vi "Calibration.vi"() -> ()   [LabVIEW 2023]
uses:
  Communication/PCAN2023/PCAN API.lvlib
panel:
  out "Read Current Offset":bool
  out "Perform Current Offset":bool
  out "Set Manifacturing":bool
  out "Nexteer Connect":bool
  out "error out":errorcluster
  in  "error in":errorcluster
  in  "Channel":u16=81 format="%x"
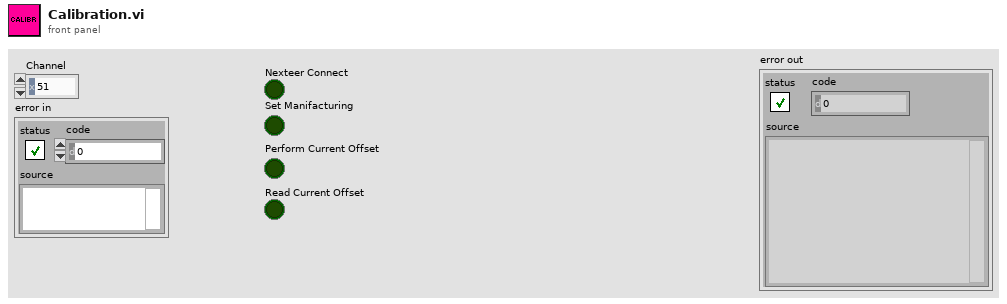
[diagram p1: front panel]
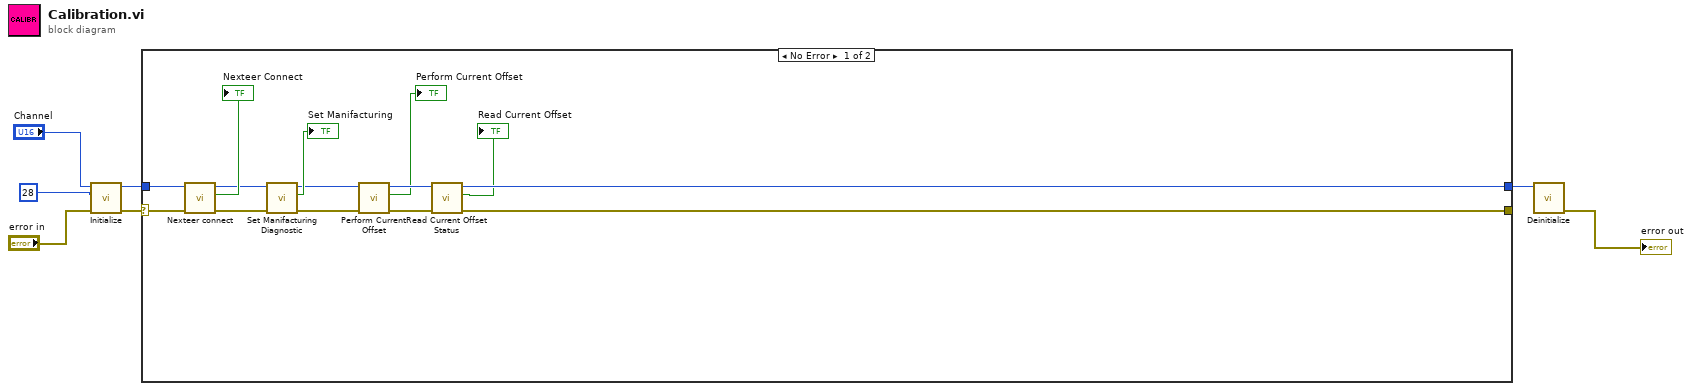
[diagram p0: block diagram]
diagram:
  n1 = call "Initialize.vi"("error in"="error in", "Btr0Btr1"=u16 28, "Channel"="Channel") -> ("error out"=w1:errorcluster, "Channel out"=w4:u16)  [unwired: 6 in, 1 out]
  n2 = case shown="No Error" w1 {
    selector: w1 -> [w20 w23]
    tunnel: w4 -> [w21 w22]
    tunnel: [w11 w22] -> w3
    tunnel: [w10 w23] -> _
    frame No Error {
      n3 = call "Nexteer connect.vi"("error in"=w20, "Channel in"=w21) -> ("error out"=w17:errorcluster, "Pass"=→"Nexteer Connect":bool, "Channel out"=w18:u16)  [unwired: 5 in]
      n4 = call "Set Manifacturing Diagnostic.vi"("error in"=w17, "Channel in"=w18) -> ("error out"=w14:errorcluster, "Pass"=→"Set Manifacturing":bool, "Channel out"=w15:u16)  [unwired: 5 in]
      n5 = call "Perform Current Offset.vi"("error in"=w14, "Channel in"=w15) -> ("error out"=w12:errorcluster, "Pass"=→"Perform Current Offset":bool, "Channel out"=w13:u16)  [unwired: 5 in]
      n6 = call "Read Current Offset Status.vi"("error in"=w12, "Channel in"=w13) -> ("error out"=w10:errorcluster, "Pass"=→"Read Current Offset":bool, "Channel out"=w11:u16)  [unwired: 5 in]
    }
    frame Error {
    }
  }
  n7 = call "Deinitialize.vi"("Channel"=w3) -> ("error out"=→"error out":errorcluster)  [unwired: 10 in]
